vi "Cursor Line Color Write.vi"(8 "error in (no error)":errorcluster, 9 "Line Color":u32(colorbox), 11 "3D Plot.lvclass in":refnum<class "3D Plot.lvclass">) -> (0 "error out":errorcluster, 3 "3D Plot.lvclass out":refnum<class "3D Plot.lvclass">)   [LabVIEW 2020, in "3D Plot.lvclass"]
uses:
  3D Plot.lvclass
  3D Plot.lvclass/3D Plot.ctl
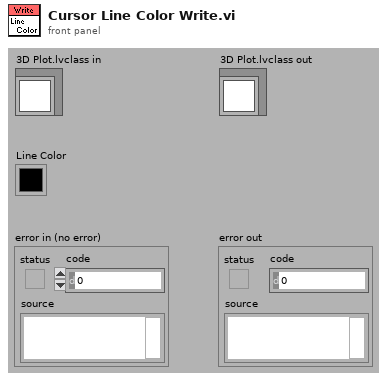
[diagram p1: front panel]
types:
  T1 = typedef "3D Plot.lvclass/Cursor Property Array.ctl" = T2[]
  T2 = typedef "3D Plot.lvclass/Cursor Property.ctl" = cluster{"Cursor Visible":bool, "Cursor Enable":bool, "Cursor Position":T3, "Cursor Point":T4, "Cursor Line":T6, "Cursor Plane":T8, "Cursor Text":T9}
  T3 = typedef "3D Plot.lvclass/Cursor Position.ctl" = cluster{"Cursor Plot ID":i32, "Cursor X":sgl, "Cursor Y":sgl, "Cursor Z":sgl, "Cursor Snap To":enum16{"Fixed", "Nearest Plot", "Snap to Plot"}}
  T4 = typedef "3D Plot.lvclass/Cursor Point.ctl" = cluster{"Cursor Point Color":u32, "Cursor Point Size":sgl, "Cursor Point Style":T5}
  T5 = typedef "3D Plot.lvclass/Sprite Type.ctl" = enum16{"None", "Empty Square", "Solid Square", "Empty Diamond", "Solid Diamond", "Empty Circle", "Solid Circle", "Asterisk", "Bold X", "Wireframe Sphere", "Solid Sphere", "Wireframe Cube", "Solid Cube"}
  T6 = typedef "3D Plot.lvclass/Cursor Line.ctl" = cluster{"Cursor Line Color":u32, "Cursor Line Width":sgl, "Cursor Line Style":T7}
  T7 = typedef "3D Plot.lvclass/Line Type.ctl" = enum16{"None", "Solid", "Dash", "Dot", "Dash Dot"}
  T8 = typedef "3D Plot.lvclass/Cursor Plane.ctl" = cluster{"Cursor Plane Color":u32, "Cursor Plane Opacity":sgl, "Draw Cursor Plane X-Z":bool, "Draw Cursor Plane Y-Z":bool, "Draw Cursor Plane X-Y":bool}
  T9 = typedef "3D Plot.lvclass/Cursor Text.ctl" = cluster{"Cursor Text":string, "Cursor Text Size":u16, "Cursor Show Position":bool, "Cursor Show Name":bool, "Cursor Text Color":u32, "Background Color":u32, "Background Opacity":sgl}
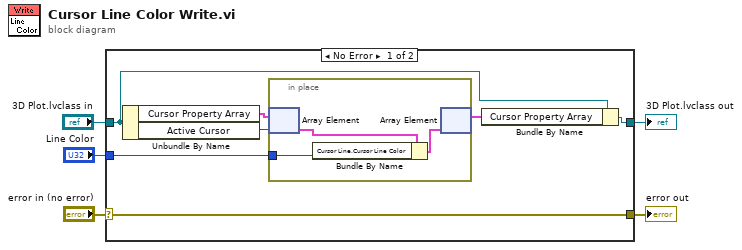
[diagram p0: block diagram]
diagram:
  n1 = case shown="No Error" "error in (no error)" {
    selector: "error in (no error)" -> [w6 w16]
    tunnel: "Line Color" -> [w12 _]
    tunnel: "3D Plot.lvclass in" -> [w8 w17]
    tunnel: [w7 w17] -> w3
    tunnel: [w6 w16] -> w1
    frame No Error {
      n2 = Unbundle By Name(w8) -> ("Cursor Property Array"=w9:T1, "Active Cursor"=w10:i32)
      n3 = in-place {
        in-place-border: w12 -> [w13]
        n4 = in-place-array #1(w9, w10) -> (w15:T2)
        n5 = Bundle By Name(cluster=w15, "Cursor Line.Cursor Line Color"=w13) -> (w14:T2)
        n6 = in-place-array #1(w14) -> (w11:T1)  [unwired: 1 out]
      }
      n7 = Bundle By Name(cluster=w8, "Cursor Property Array"=w11) -> (w7:refnum<class "3D Plot.lvclass">)
    }
    frame Error {
    }
  }
  "error out" <- w1
  "3D Plot.lvclass out" <- w3
